vi "Get Double.vi"(8 "error in (no error)":errorcluster, 11 "DblMessage In":refnum<class "DblMessage.lvclass">) -> (0 "error out":errorcluster, 2 "Message Data":dbl, 3 "DblMessage Out":refnum<class "DblMessage.lvclass">)   [LabVIEW 2009, in "LapDog.Messaging.v2.NativeTypes.lvlib" / "DblMessage.lvclass"]
doc: "Returns the data contained in the message.\n\nThis method executes regardless of the error in state."
uses:
  DblMessage.lvclass
  DblMessage.lvclass/DblMessage.ctl
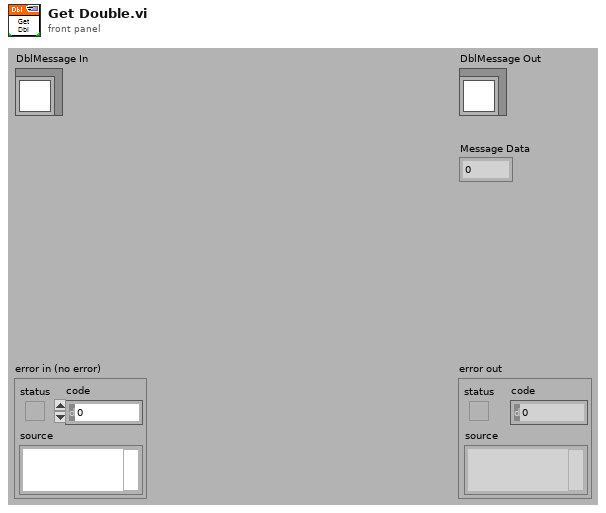
[diagram p1: front panel]
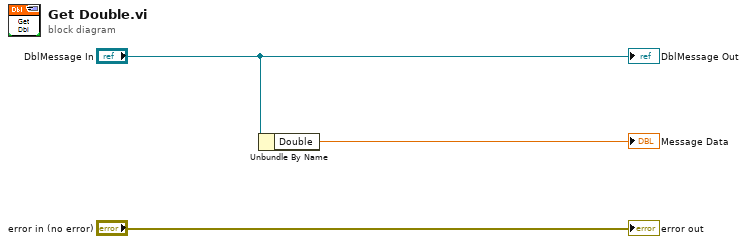
[diagram p0: block diagram]
diagram:
  n1 = Unbundle By Name("DblMessage In") -> ("Double"=→"Message Data":dbl)
  "error out" <- "error in (no error)"
  "DblMessage Out" <- "DblMessage In"
